vi "DSF.Engine.Framework.Error Handler.Check for Transceiver Errors.vi"(8 "error in (no error)":errorcluster, 11 "Framework in":refnum<class "DSF.Engine.Framework.lvclass">) -> (0 "error out":errorcluster, 3 "Framework out":refnum<class "DSF.Engine.Framework.lvclass">)   [LabVIEW 2017, in "Data Sharing Framework Engine.lvlib" / "DSF.Engine.Framework.lvclass"]
uses:
  DSF.Engine.Framework.lvclass
  DSF.Engine.Framework.lvclass/DSF.Engine.Framework.ctl
  Plugin/DSF.Engine.Plugin.lvclass/DSF.Engine.Plugin.ctl
  Source/Data Sharing Framework Core/Engine/Interfaces/Transceiver Interface/Read Transceiver Error.vi
  Plugin/DSF.Engine.Plugin.lvclass
  Source/Data Sharing Framework Core/Engine/Interfaces/Transceiver Interface/Transceiver Interface.lvclass
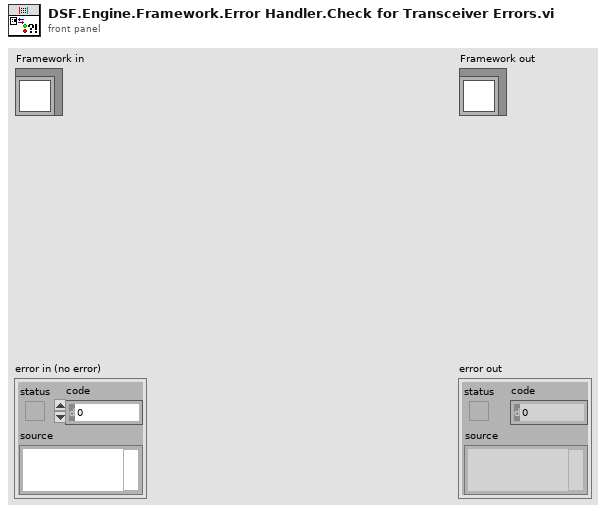
[diagram p1: front panel]
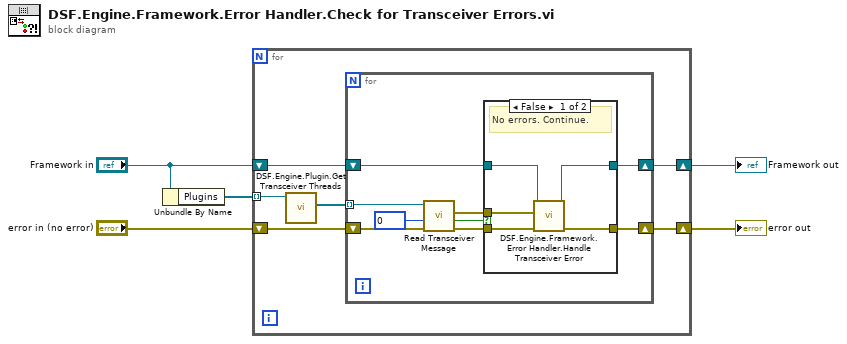
[diagram p0: block diagram]
diagram:
  n1 = Unbundle By Name("Framework in") -> ("Plugins"=w3:refnum<class "DSF.Engine.Plugin.lvclass">[])
  n2 = for {
    tunnel: w3 -> [w11] mode=indexing
    shift-right: [w8] -> w4
    shift-left: "error in (no error)" -> [w9]
    shift-right: [w6] -> w1
    shift-left: "Framework in" -> [w7]
    n3 = call "DSF.Engine.Plugin.Get Transceiver Threads.vi"("Plugin in"=w11) -> ("Transceiver Threads"=w10:refnum<class "Transceiver Interface.lvclass">[])  [unwired: 9 in, 1 out]
    n4 = for {
      tunnel: w10 -> [w20] mode=indexing
      shift-right: [w14] -> w8
      shift-left: w9 -> [w19]
      shift-right: [w12] -> w6
      shift-left: w7 -> [w13]
      n5 = call-poly "Read Transceiver Message.vi"("error in (no error)"=w19, "timeout in ms (0)"=0, "Transceiver Interface in"=w20) -> ("error out"=w15:errorcluster, "empty?"=w17:bool, "error"=w16:errorcluster)  [unwired: 5 in, 1 out]
      n6 = case shown="False" w17 {
        tunnel: w16 -> [w21 _]
        tunnel: w15 -> [w23 w27]
        tunnel: [w22 w27] -> w14
        tunnel: w13 -> [w25 w26]
        tunnel: [w24 w26] -> w12
        frame False {
          # "No errors. Continue."
          n7 = call "DSF.Engine.Framework.Error Handler.Handle Transceiver Error.vi"("error in (no error)"=w23, "transceiver error"=w21, "Framework in"=w25) -> ("error out"=w22:errorcluster, "Framework out"=w24:refnum<class "DSF.Engine.Framework.lvclass">)  [unwired: 7 in]
        }
        frame True {
          # "Incoming thread error. Handle."
        }
      }
    }
  }
  "error out" <- w4
  "Framework out" <- w1
